vi "calculate_p_hat_parallel.vi"(8 "Error In":errorcluster, 9 "m":dbl, 10 "xi":dbl, 11 "gamma":dbl) -> (0 "Error Out":errorcluster, 3 "p hat parallel":dbl[](array[numeric]))   [LabVIEW 2019]
doc: "Calculate phi from formula 4 in Wilen(2000). All inputs and outputs are in degrees."
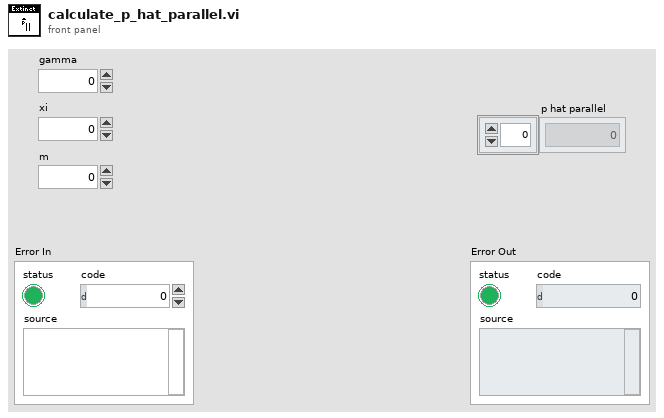
[diagram p1: front panel]
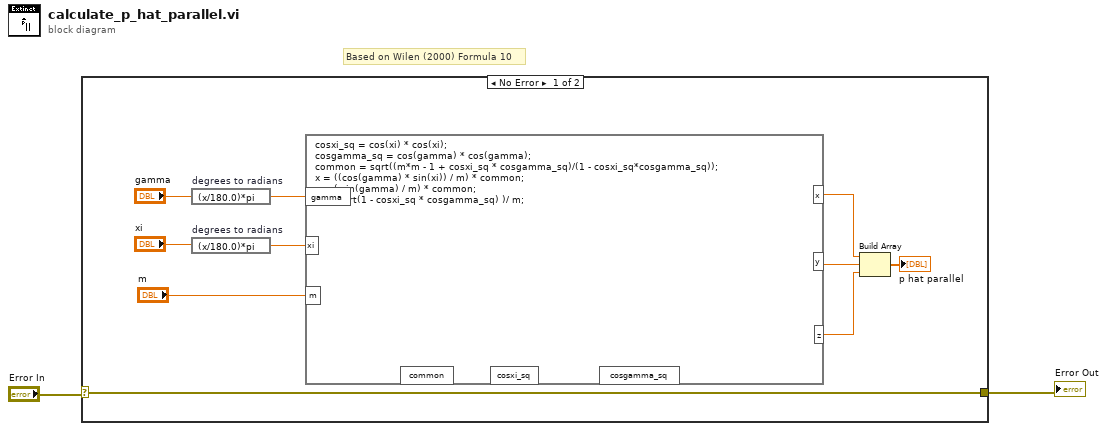
[diagram p0: block diagram]
diagram:
  # "Based on Wilen (2000) Formula 10"
  n1 = case shown="No Error" "Error In" {
    selector: "Error In" -> [w12 w13]
    tunnel: [w12 w13] -> w1
    frame No Error {
      n2 = expression code="(x/180.0)*pi" "degrees to radians"("gamma") -> (w11:dbl)
      n3 = expression code="(x/180.0)*pi" "degrees to radians"("xi") -> (w10:dbl)
      n4 = formula code="cosxi_sq = cos(xi) * cos(xi);\ncosgamma_sq = cos(gamma) * cos(gamma);\ncommon = sqrt((m*m - 1 + cosxi_sq * cosgamma_sq)/(1 - cosxi_sq*cosgamma_sq));\nx = ((cos(gamma) * sin(xi)) / m) * common;\ny = (-sin(gamma) / m) * common;\nz = (sqrt(1 - cosxi_sq * cosgamma_sq) )/ m;"("gamma"=w11, "xi"=w10, "m"="m") -> ("x"=w6:dbl, "y"=w7:dbl, "z"=w5:dbl)  [unwired: 3 out]
      n5 = Build Array(w6, w7, w5) -> (→"p hat parallel":dbl[])
    }
    frame Error {
    }
  }
  "Error Out" <- w1
